vi "ProbeStationAutomation.vi"() -> ()   [LabVIEW 2020]
uses:
  Control 2.ctl
  C:/Users/User/Desktop/Automation/CurrentVersion/LabviewDXFViewer/bin/Release/LabviewDXFViewer.exe
  LabviewDXFViewer/bin/Release/LabviewDXFViewer.exe
  UIReferences.ctl
  WaferAlignmentType.ctl
  <vilib>/Utility/file.llb/Write Delimited Spreadsheet (DBL).vi
  Keithley 2600 Series/Keithley 2600 Series.lvlib
panel:
  in  "StartOxide":refnum<k24>(container)
  out "WaferAlignment":T1
  out "UiDefinition 3":T2
  in  "PathInfos":T3
  in  "UiDefinition 2":T2
  out "SweepInfo":T4
  out "error out":errorcluster
  out "Position 3":i32[](array[numeric])
  out "Position 2":i32[](array[numeric])
  out "Status":string="Please Load/Select probe site list"
  in  "Chip Orientation":i32(ring) items=["Horizontal", "Vertical"]
  in  "TextEditor":refnum<k24>(container)
  out "WaferTestPoints":string
  out "TestPointsLoaded":bool
  out "dxfFile":string
  out "error out 5":errorcluster
  out "Fit Array":string[][](array[string])
  out "error out 4":errorcluster
  out "error out 3":errorcluster
  out "Fit":dbl[][](array[numeric])
  out "IV Scan Data":dbl[][](array[numeric])
  out "Rotation Misalign":dbl[](array[numeric])
  out "Scale Misalign":dbl
  out "Position 1":i32[](array[numeric])
  in  "Microsites":refnum<k24>(container)
  in  "DXFCanvas":refnum<k24>(container)
  in  "WebCamViewer":refnum<k24>(container)
  in  "IV Curves":T5
  in  "Tab Control":T6(tab)
  in  "ClearPositions":bool
  in  "User":string
  in  "resetcontact":bool
  in  "EnableJoystick":bool
  in  "StartCycle":refnum<k24>(container)
  in  "Version":string
  in  "Experiment":string
  in  "Lower":refnum<k24>(container)
  in  "Raise":refnum<k24>(container)
  in  "West":refnum<k24>(container)
  in  "East":refnum<k24>(container)
  in  "North":refnum<k24>(container)
  in  "South":refnum<k24>(container)
  in  "Align Position 1":bool
  in  "Platten Move":refnum<k24>(container)
  in  "Masks":string(combo)
  in  "Move Position 1":bool
  in  "Align Position 3":bool
  in  "Position 3":bool
  in  "Align Position 2":bool
  in  "Position 2":bool
  in  "Die":string
  in  "Wafer":string
  in  "Jog (um) 2":dbl=100.0
  in  "Jog (um)":dbl=500.0
  in  "Load Mask":bool
  in  "Save Wafer":bool
  in  "Lift Distance (um)":dbl=2000.0
  in  "Quit":bool
  out "In Contact":bool
  out "Motor Position":string
  in  "Save Tag":string
  out "Capacitance":dbl
  in  "Current Range (A)":dbl=1e-10
  in  "Junction":string(combo)="None"
  in  "Sweeps":dbl=2.0
  in  "Number Points":dbl=200.0
  in  "Minimum (mV)":dbl=-100.0
  in  "Maxiumum (mV)":dbl=100.0
  in  "Source Measure Unit Channel (0: Channel A)":i32(ring) items=["Channel A", "Channel B"]
  in  "VISA resource name":refnum<visa-resource-name>="Keithley_2636A"
  in  "Scan":bool
  in  "Save Scan":bool
  out "Conductance":dbl
  out "Intercept":dbl
  out "XY Graph":cluster{"x":timestamp, "y":dbl}[](graph)
  in  "Steps Per micron":dbl=0.629
  in  "Stepper Controller Port":i32=3
  out "GetCameras":string[](array[string])
  in  "Wafer Definition File":path=path "C:/Users/User/Desktop/Automation/ASU FG Mask 21.08.26.dxf"
  in  "Wafer Units to microns":dbl=1.0
  in  "Data Path":path=path "C:/Users/User/Desktop/Automation/data"
  # "Run Oxide"
  # "Optional Tags"
  # "Jog Platten"
  # "Platten Altitude"
  # "Run IVs"
  # "Cycle Step"
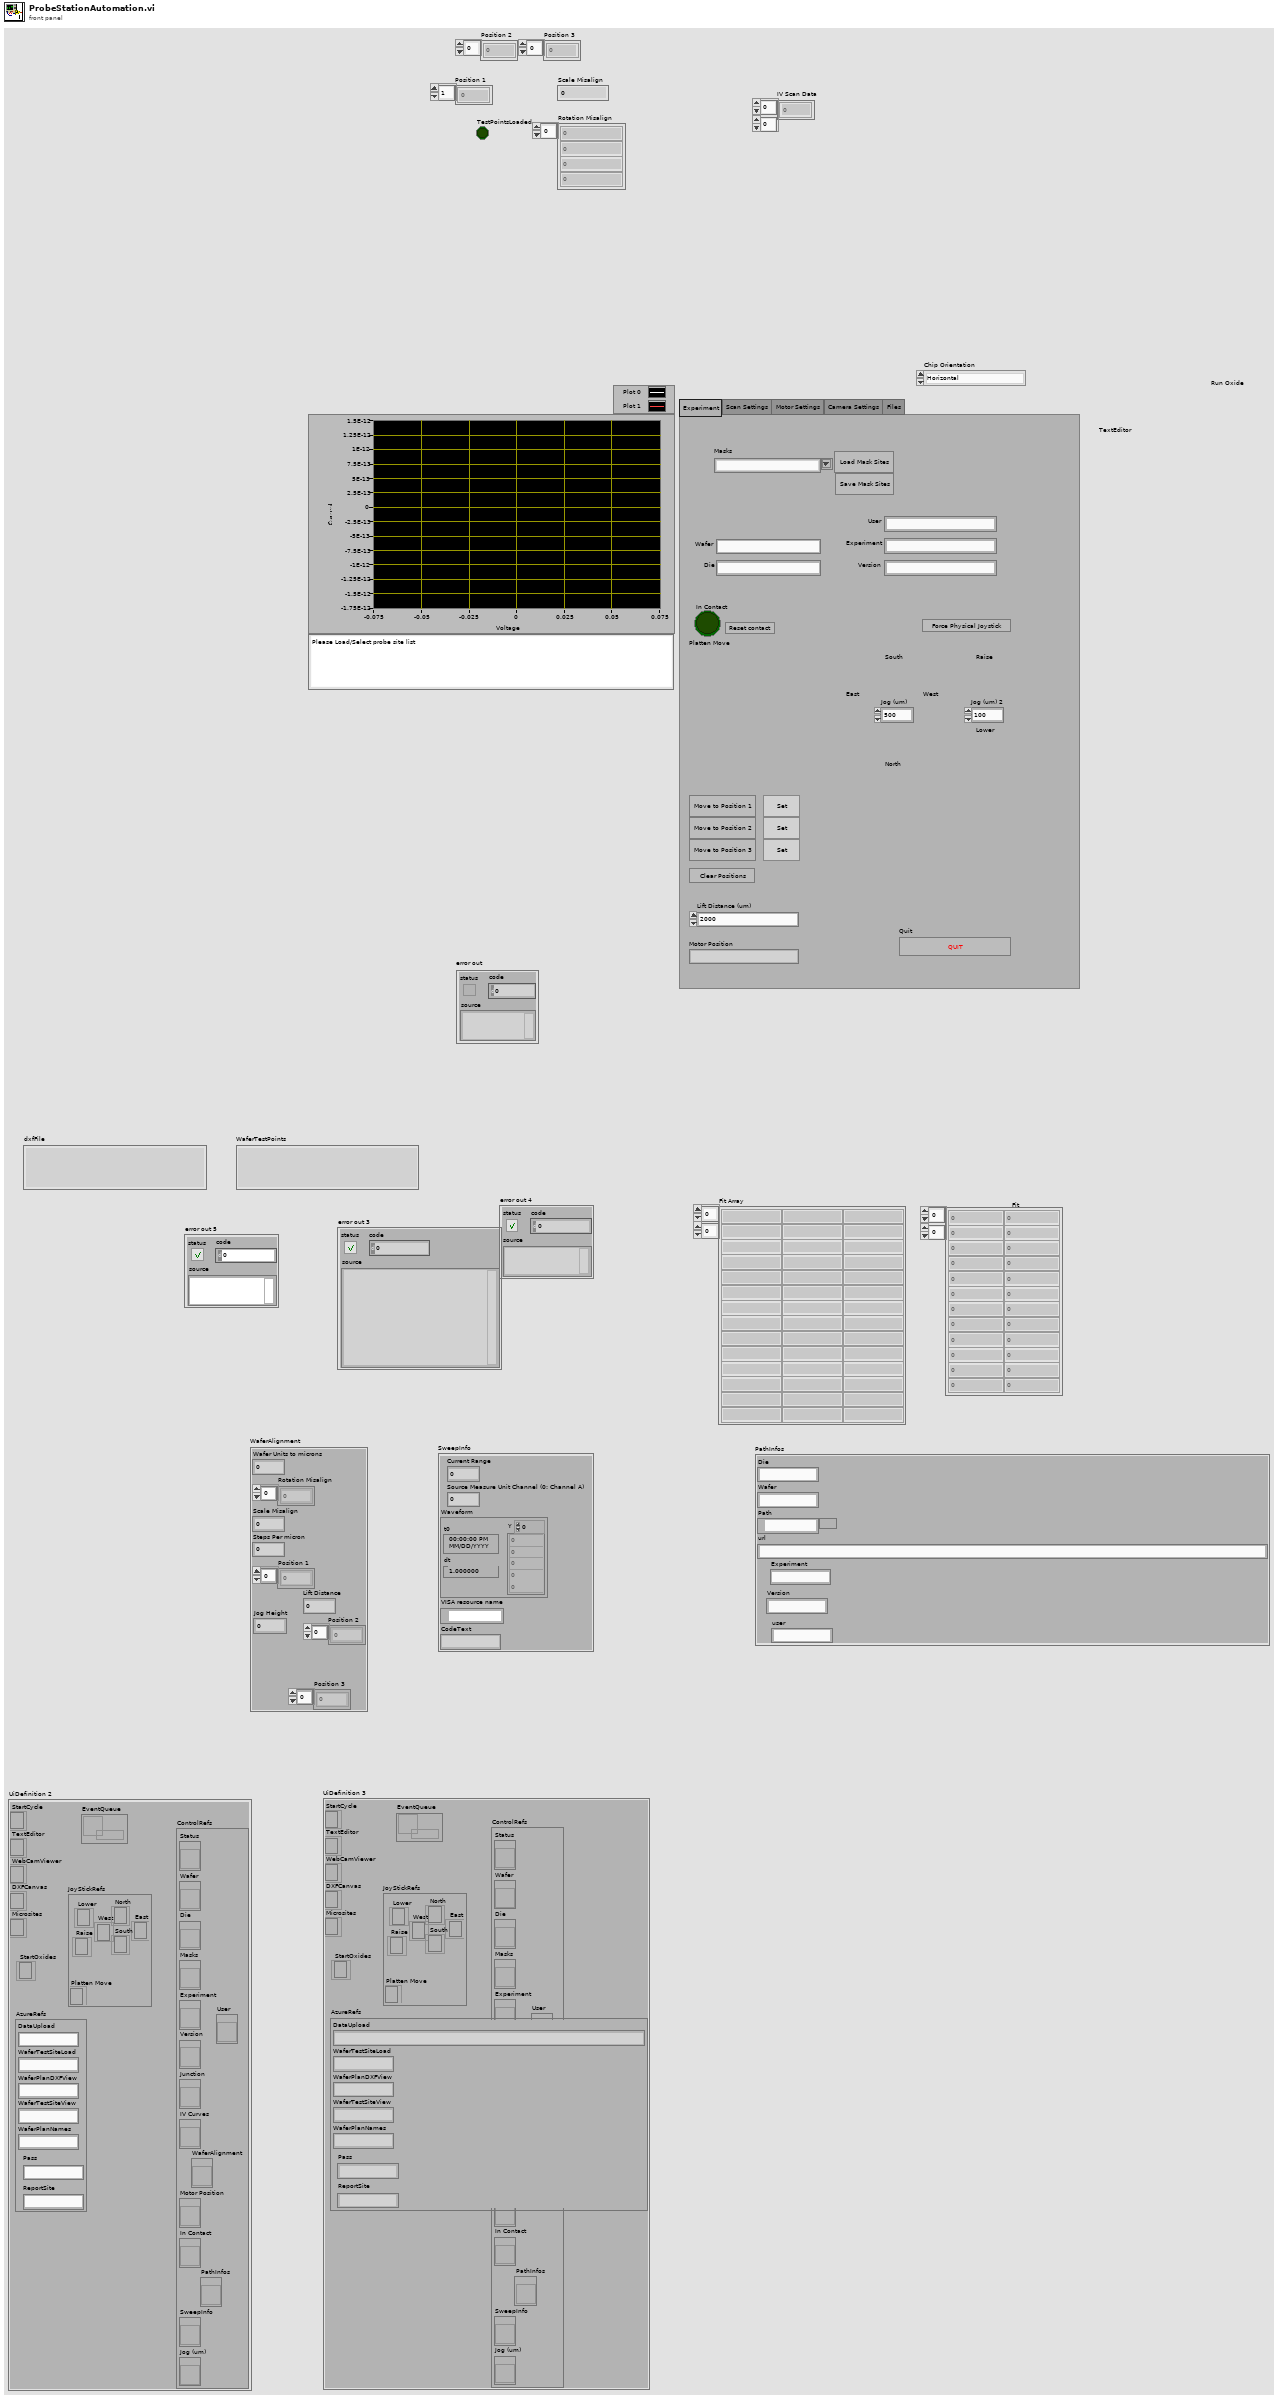
[diagram p1: front panel]
types:
  T1 = typedef "WaferAlignmentType.ctl" = cluster{"Wafer Units to microns":dbl, "Rotation Misalign":dbl[], "Scale Misalign":dbl, "Steps Per micron":dbl, "Position 1":i32[], "Position 2":i32[], "Lift Distance":i32, "Position 3":i32[], "Jog Height":i32}
  T2 = typedef "UIReferences.ctl" = cluster{"StartCycle":refnum<k24>, "TextEditor":refnum<k24>, "WebCamViewer":refnum<k24>, "DXFCanvas":refnum<k24>, "Microsites":refnum<k24>, "JoyStickRefs":cluster{"North":refnum<k24>, "Lower":refnum<k24>, "Raise":refnum<k24>, "Platten Move":refnum<k24>, "West":refnum<k24>, "East":refnum<k24>, "South":refnum<k24>}, "AzureRefs":cluster{"DataUpload":string, "WaferTestSiteLoad":string, "WaferPlanDXFView":string, "WaferTestSiteView":string, "WaferPlanNames":string, "Pass":string, "ReportSite":string}, "ControlRefs":cluster{"Status":refnum<vi>, "Wafer":refnum<vi>, "Die":refnum<vi>, "Masks":refnum<vi>, "Experiment":refnum<vi>, "Version":refnum<vi>, "Junction":refnum<vi>, "IV Curves":refnum<vi>, "Motor Position":refnum<vi>, "In Contact":refnum<vi>, "SweepInfo":refnum<vi>, "Jog (um)":refnum<vi>, "PathInfos":refnum<vi>, "User":refnum<vi>, "WaferAlignment":refnum<vi>}, "EventQueue":refnum<queue>, "StartOxides":refnum<k24>}
  T3 = cluster{"Die":string, "Wafer":string, "Path":path, "url":string, "Experiment":string, "Version":string, "user":string}
  T4 = cluster{"Current Range":dbl, "Source Measure Unit Channel (0: Channel A)":i32, "Waveform":waveform(dbl), "VISA resource name":refnum<visa-resource-name>, "CodeText":string}
  T5 = typedef "Control 2.ctl" = cluster{"Y":dbl[], "Current (A)":dbl[]}
  T6 = enum32{"Experiment", "Scan Settings", "Motor Settings", "Camera Settings", "Files"}
  T7 = cluster{"DataUpload":string, "WaferTestSiteLoad":string, "WaferPlanDXFView":string, "WaferTestSiteView":string, "WaferPlanNames":string, "Pass":string, "ReportSite":string}
  T8 = cluster{"North":refnum<k24>, "Lower":refnum<k24>, "Raise":refnum<k24>, "Platten Move":refnum<k24>, "West":refnum<k24>, "East":refnum<k24>, "South":refnum<k24>}
  T9 = cluster{"Status":refnum<vi>, "Wafer":refnum<vi>, "Die":refnum<vi>, "Masks":refnum<vi>, "Experiment":refnum<vi>, "Version":refnum<vi>, "Junction":refnum<vi>, "IV Curves":refnum<vi>, "Motor Position":refnum<vi>, "In Contact":refnum<vi>, "SweepInfo":refnum<vi>, "Jog (um)":refnum<vi>, "PathInfos":refnum<vi>, "User":refnum<vi>, "WaferAlignment":refnum<vi>}
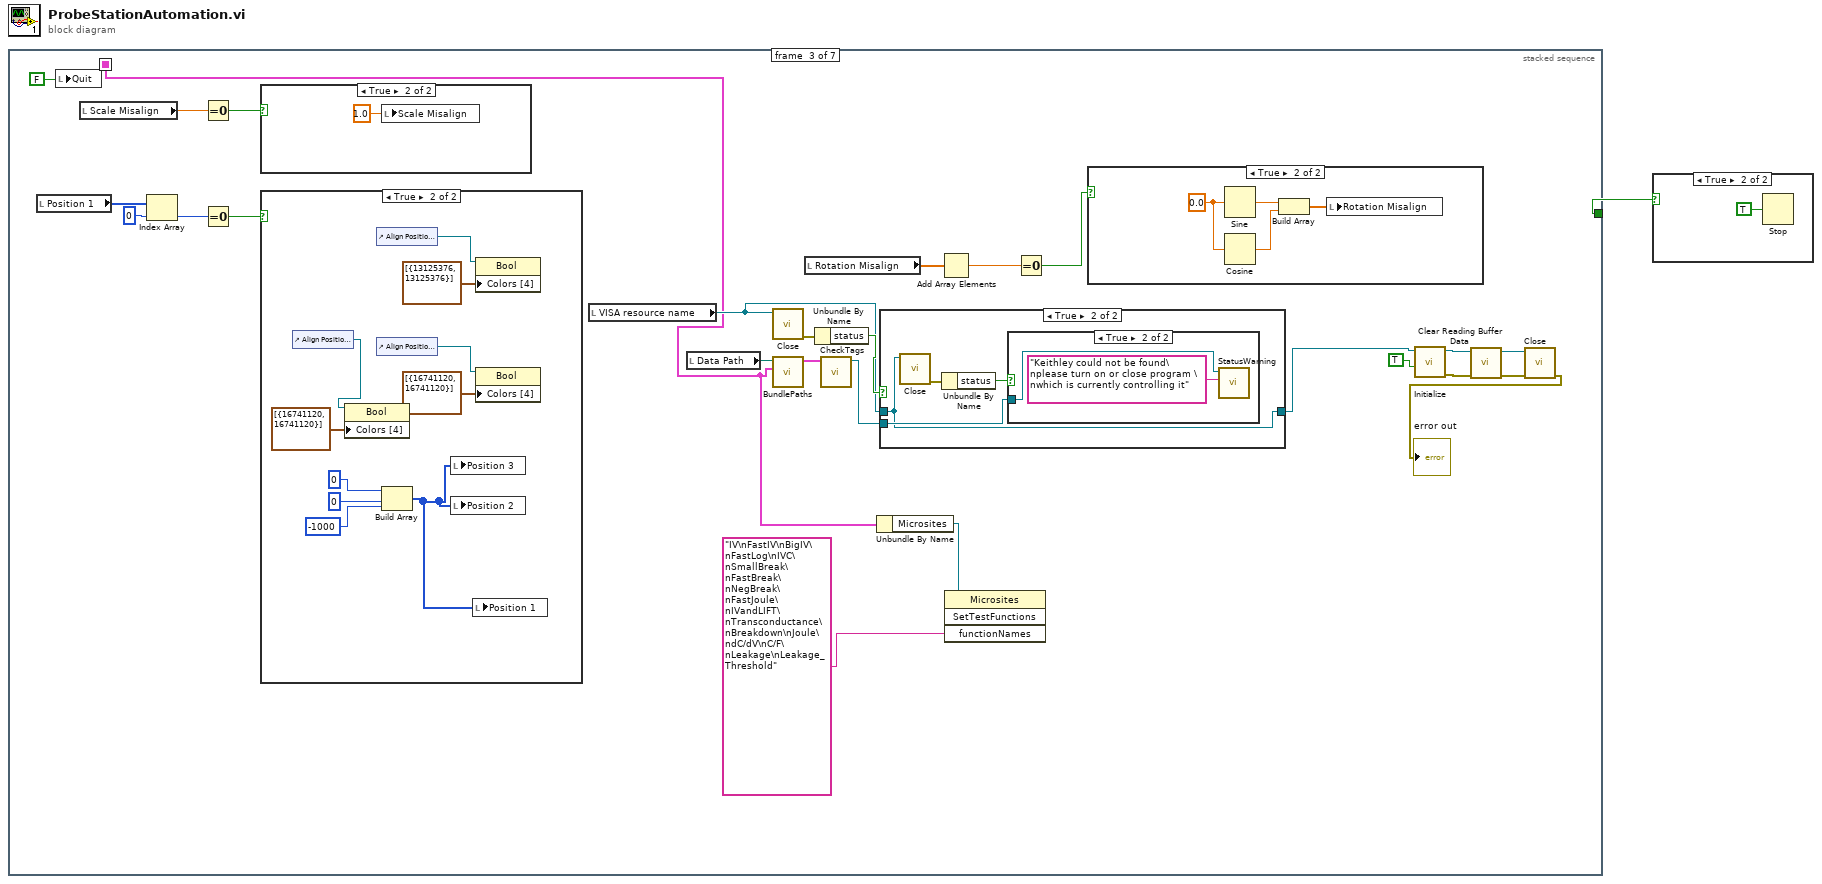
[diagram p0: block diagram]
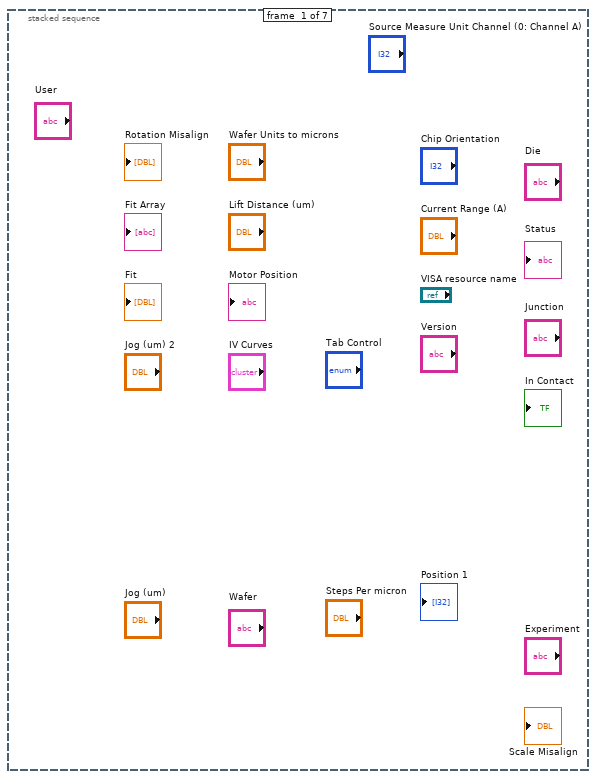
[diagram p3: hidden frame]
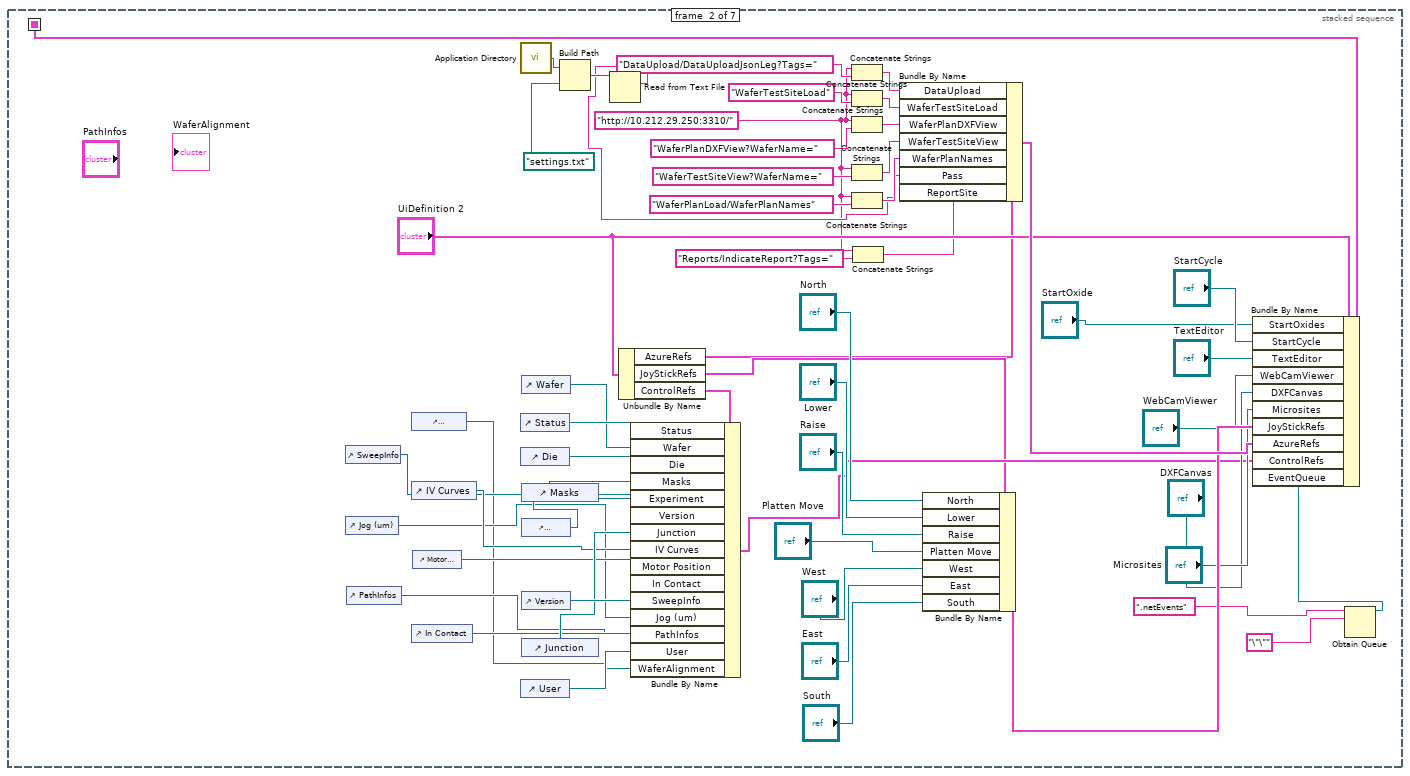
[diagram p4: hidden frame]
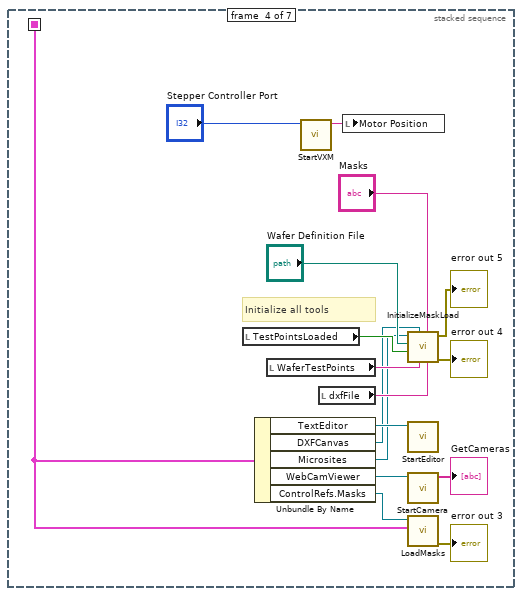
[diagram p10: hidden frame]
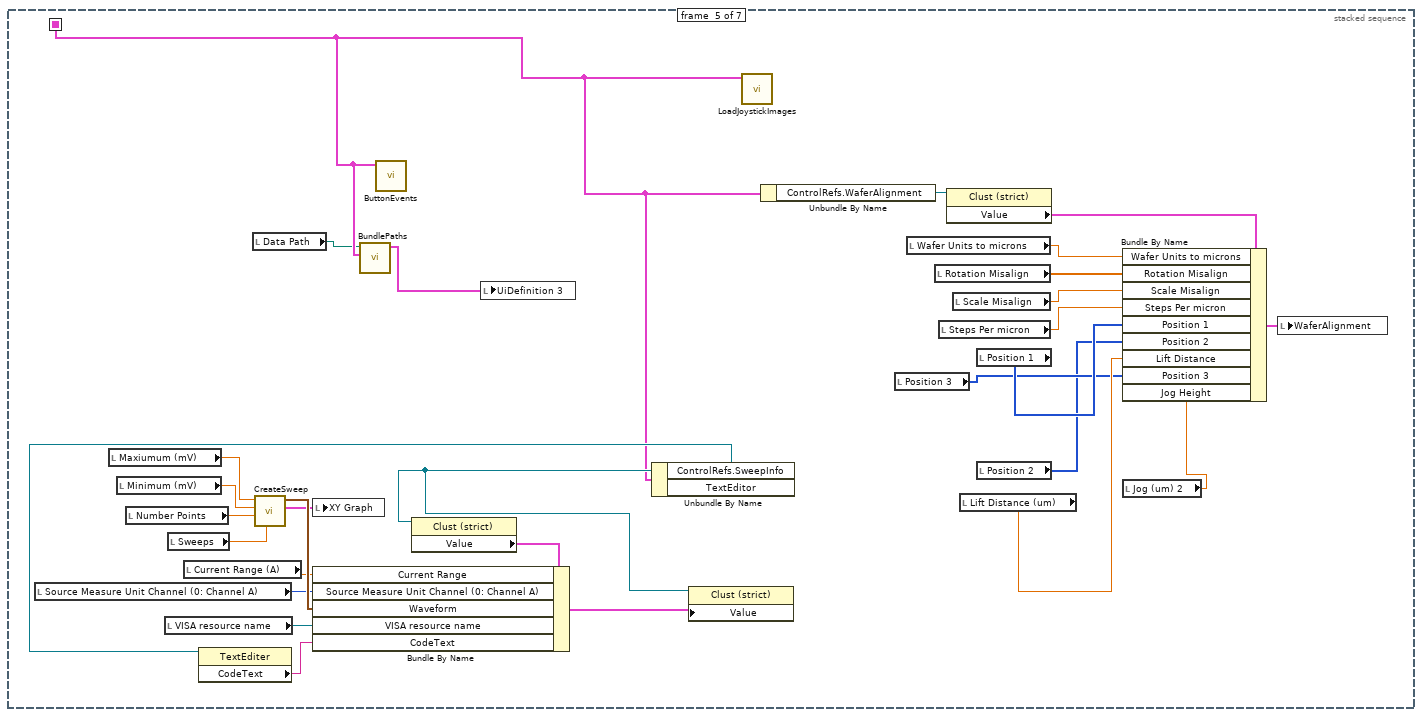
[diagram p11: hidden frame]
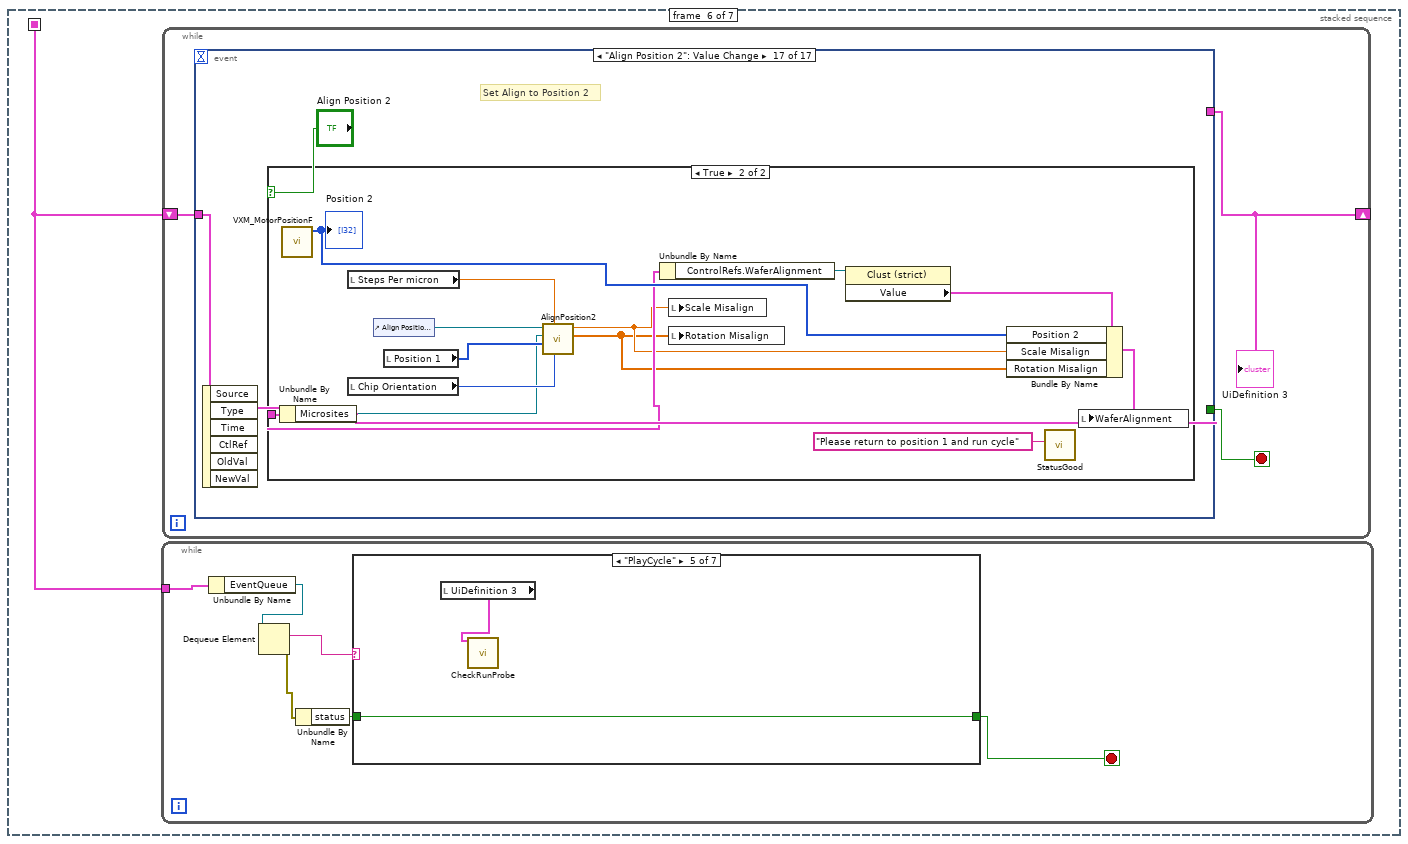
[diagram p12: hidden frame]
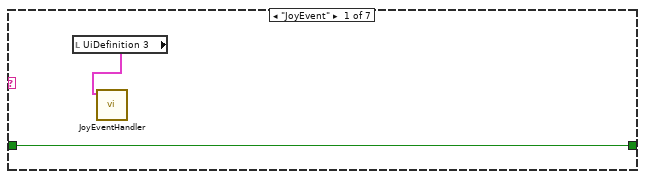
[diagram p13: hidden frame]
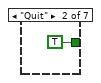
[diagram p14: hidden frame]
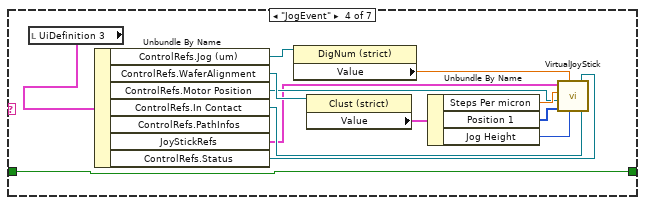
[diagram p16: hidden frame]
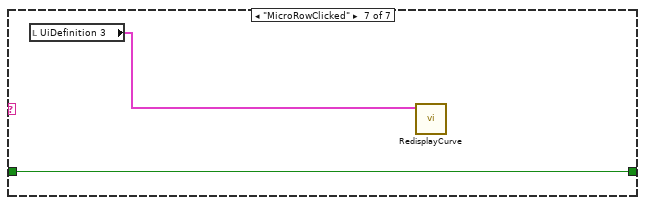
[diagram p18: hidden frame]
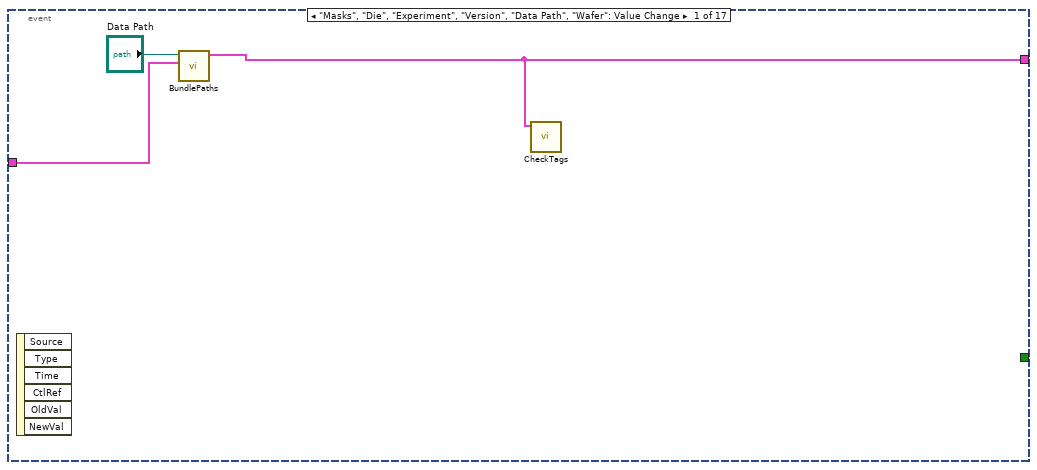
[diagram p19: hidden frame]
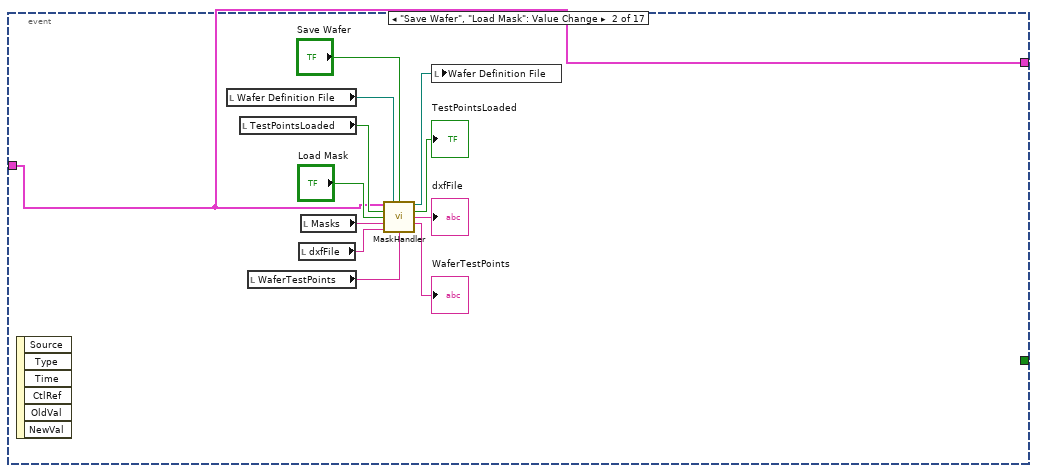
[diagram p20: hidden frame]
diagram:
  n1 = stacked-sequence {
    seq-local: [_ w44 _ _ _ _ _] -> [_ _ w60 w106 w125 w152 _]
    tunnel: [_ _ _ _ _ _ TRUE ("Quit")] -> w1
    frame #0 {
    }
    frame #1 {
      w3 = "http://10.212.29.250:3310/"
      n2 = control-ref of="SweepInfo"() -> (w29:refnum<vi>)
      n3 = control-ref of="Jog (um)"() -> (w28:refnum<vi>)
      n4 = control-ref of="PathInfos"() -> (w27:refnum<vi>)
      n5 = control-ref of="WaferAlignment"() -> (w5:refnum<vi>)
      n6 = control-ref of="IV Curves"() -> (w32:refnum<vi>)
      n7 = control-ref of="In Contact"() -> (w30:refnum<vi>)
      n8 = control-ref of="Motor Position"() -> (w31:refnum<vi>)
      n9 = call <vilib>:"Application Directory.vi"() -> ("Application Directory"=w8:path)
      n10 = control-ref of="Status"() -> (w39:refnum<vi>)
      n11 = control-ref of="Die"() -> (w37:refnum<vi>)
      n12 = control-ref of="User"() -> (w22:refnum<vi>)
      n13 = control-ref of="Wafer"() -> (w38:refnum<vi>)
      n14 = control-ref of="Masks"() -> (w36:refnum<vi>)
      n15 = control-ref of="Experiment"() -> (w35:refnum<vi>)
      n16 = control-ref of="Version"() -> (w34:refnum<vi>)
      n17 = control-ref of="Junction"() -> (w33:refnum<vi>)
      n18 = Build Path(base path=w8, name or relative path=path "settings.txt" ("file (use dialog)")) -> (appended path=w10:path)
      n19 = Read from Text File(file (use dialog)=w10) -> (text=w7:string)  [unwired: 3 in, 3 out]
      n20 = Unbundle By Name("UiDefinition 2") -> ("AzureRefs"=w21:T7, "JoyStickRefs"=w26:T8, "ControlRefs"=w41:T9)
      n21 = Bundle By Name(cluster=w41, "Status"=w39, "Wafer"=w38, "Die"=w37, "Masks"=w36, "Experiment"=w35, "Version"=w34, "Junction"=w33, "IV Curves"=w32, "Motor Position"=w31, "In Contact"=w30, "SweepInfo"=w29, "Jog (um)"=w28, "PathInfos"=w27, "User"=w22, "WaferAlignment"=w5) -> (w40:T9)
      n22 = Concatenate Strings(w3, "DataUpload/DataUploadJsonLeg?Tags=" ("url")) -> (w20:string)
      n23 = Concatenate Strings(w3, "WaferTestSiteLoad" ("url")) -> (w17:string)
      n24 = Concatenate Strings(w3, "WaferPlanDXFView?WaferName=" ("url")) -> (w15:string)
      n25 = Concatenate Strings(w3, "WaferTestSiteView?WaferName=" ("url")) -> (w13:string)
      n26 = Concatenate Strings(w3, "WaferPlanLoad/WaferPlanNames" ("url")) -> (w11:string)
      n27 = Concatenate Strings(w3, "Reports/IndicateReport?Tags=" ("string")) -> (w4:string)
      n28 = Bundle By Name(cluster=w21, "DataUpload"=w20, "WaferTestSiteLoad"=w17, "WaferPlanDXFView"=w15, "WaferTestSiteView"=w13, "WaferPlanNames"=w11, "Pass"=w7, "ReportSite"=w4) -> (w57:T7)
      n29 = Bundle By Name(cluster=w26, "North"="North", "Lower"="Lower", "Raise"="Raise", "Platten Move"="Platten Move", "West"="West", "East"="East", "South"="South") -> (w53:T8)
      n30 = Obtain Queue(name (unnamed)=".netEvents", element data type="\"\"") -> (queue out=w23:refnum<queue>)  [unwired: 3 in, 2 out]
      n31 = Bundle By Name(cluster="UiDefinition 2", "StartOxides"="StartOxide", "StartCycle"="StartCycle", "TextEditor"="TextEditor", "WebCamViewer"="WebCamViewer", "DXFCanvas"="DXFCanvas", "Microsites"="Microsites", "JoyStickRefs"=w53, "AzureRefs"=w57, "ControlRefs"=w40, "EventQueue"=w23) -> (w44:T2)
    }
    frame #2 {
      n32 = local read "Position 1"() -> (w82:i32[])
      n33 = local write "Quit"(FALSE) -> ()
      n34 = local read "Scale Misalign"() -> (w77:dbl)
      n35 = Index Array(array=w82, index=0) -> (element=w83:i32)
      n36 = Equal To 0?(x=w77) -> (x = 0?=w76:bool)
      n37 = Equal To 0?(x=w83) -> (x = 0?=w81:bool)
      n38 = case shown="True" w76 {
        frame False {
        }
        frame True {
          n39 = local write "Scale Misalign"(1.0 ("Scale Misalign")) -> ()
        }
      }
      n40 = case shown="True" w81 {
        frame False {
        }
        frame True {
          n41 = control-ref of="Align Position 3"() -> (w91:refnum<vi>)
          n42 = property class="Bool"(reference=w91, "Colors [4]"=cluster{u32, u32}[] [{16741120, 16741120}]) -> ()  [unwired: 1 in, 2 out]
          n43 = control-ref of="Align Position 1"() -> (w100:refnum<vi>)
          n44 = control-ref of="Align Position 2"() -> (w98:refnum<vi>)
          n45 = Build Array(0 ("Y"), 0 ("X"), -1000) -> (w93:i32[])
          n46 = local write "Position 3"(w93) -> ()
          n47 = local write "Position 2"(w93) -> ()
          n48 = local write "Position 1"(w93) -> ()
          n49 = property class="Bool"(reference=w100, "Colors [4]"=cluster{u32, u32}[] [{13125376, 13125376}]) -> ()  [unwired: 1 in, 2 out]
          n50 = property class="Bool"(reference=w98, "Colors [4]"=cluster{u32, u32}[] [{16741120, 16741120}]) -> ()  [unwired: 1 in, 2 out]
        }
      }
      n51 = local read "VISA resource name"() -> (w69:refnum<visa-resource-name>)
      n52 = local read "Data Path"() -> (w66:path)
      n53 = call "Close.vi"("VISA resource name"=w69) -> ("error out"=w73:errorcluster)  [unwired: 10 in]
      n54 = call "BundlePaths.vi"("Data Path"=w66, "UiDefinition 2"=w60) -> ("UiDefinition 3"=w67:T2)  [unwired: 8 in]
      n55 = local read "Rotation Misalign"() -> (w80:dbl[])
      n56 = Unbundle By Name(w73) -> ("status"=w72:bool)
      n57 = call "CheckTags.vi"("UiDefinition 2"=w67) -> ("StatusOut"=w71:refnum<vi>)  [unwired: 10 in]
      n58 = Unbundle By Name(w60) -> ("Microsites"=w59:refnum<k24>)
      n59 = case shown="True" w72 {
        tunnel: w71 -> [_ w88]
        tunnel: w69 -> [w84 w87]
        tunnel: [w84 w87] -> w68
        frame False {
        }
        frame True {
          n60 = call "Close.vi"("VISA resource name"=w87) -> ("error out"=w86:errorcluster)  [unwired: 10 in]
          n61 = Unbundle By Name(w86) -> ("status"=w85:bool)
          n62 = case shown="True" w85 {
            tunnel: w88 -> [_ w89]
            frame False {
            }
            frame True {
              n63 = call "StatusWarning.vi"("Text.Text"="Keithley could not be found\nplease turn on or close program \nwhich is currently controlling it", "String in"=w89) -> ()  [unwired: 10 in]
            }
          }
        }
      }
      n64 = Add Array Elements(numeric array=w80) -> (sum=w79:dbl)
      n65 = invoke class="Microsites" method="SetTestFunctions"(reference=w59, "functionNames"="IV\nFastIV\nBigIV\nFastLog\nIVC\nSmallBreak\nFastBreak\nNegBreak\nFastJoule\nIVandLIFT\nTransconductance\nBreakdown\nJoule\ndC/dV\nC/F\nLeakage\nLeakage_Threshold") -> ()  [unwired: 2 in, 4 out]
      n66 = Equal To 0?(x=w79) -> (x = 0?=w78:bool)
      n67 = case shown="True" w78 {
        frame False {
        }
        frame True {
          w101 = 0.0 ("x")
          n68 = Sine(x=w101) -> (sin(x)=w104:dbl)
          n69 = Cosine(x=w101) -> (cos(x)=w103:dbl)
          n70 = Build Array(w104, w103) -> (w102:dbl[])
          n71 = local write "Rotation Misalign"(w102) -> ()
        }
      }
      n72 = call "Initialize.vi"("Reset (True)"=TRUE, "VISA resource name"=w68) -> ("error out"=w64:errorcluster, "VISA resource name out"=w65:refnum<visa-resource-name>)  [unwired: 8 in]
      n73 = call "Clear Reading Buffer Data.vi"("error in (no error)"=w64, "VISA resource name"=w65) -> ("error out"=w63:errorcluster, "VISA resource name out"=w62:refnum<visa-resource-name>)  [unwired: 8 in]
      n74 = call "Close.vi"("error in (no error)"=w63, "VISA resource name"=w62) -> ("error out"=→"error out":errorcluster)  [unwired: 9 in]
    }
    frame #3 {
      # "Initialize all tools"
      n75 = local read "TestPointsLoaded"() -> (w117:bool)
      n76 = Unbundle By Name(w106) -> ("TextEditor"=w111:refnum<k24>, "DXFCanvas"=w110:refnum<k24>, "Microsites"=w109:refnum<k24>, "WebCamViewer"=w108:refnum<k24>, "ControlRefs.Masks"=w107:refnum<vi>)
      n77 = local read "WaferTestPoints"() -> (w116:string)
      n78 = call "StartVXM.vi"("Stepper Controller Port"="Stepper Controller Port") -> ("String"=w112:string)  [unwired: 10 in]
      n79 = local read "dxfFile"() -> (w115:string)
      n80 = local write "Motor Position"(w112) -> ()
      n81 = call "InitializeMaskLoad.vi"("dxfFile"=w115, "Masks"="Masks", "WaferTestPoints"=w116, "DXFCanvas"=w110, "TestPointsLoaded"=w117, "Wafer Definition File"="Wafer Definition File", "MicrositesRef"=w109) -> ("error out"=→"error out 4":errorcluster, "error out 5"=→"error out 5":errorcluster)  [unwired: 3 in]
      n82 = call "StartEditor.vi"("CodeEditorRef"=w111) -> ()  [unwired: 11 in]
      n83 = call "StartCamera.vi"("WebCamViewerRef"=w108) -> ("GetCameras"=→"GetCameras":string[])  [unwired: 10 in]
      n84 = call "LoadMasks.vi"("UiDefinition 2"=w106, "ComboBox in"=w107) -> ("error out"=→"error out 3":errorcluster)  [unwired: 9 in]
    }
    frame #4 {
      n85 = local read "Source Measure Unit Channel (0: Channel A)"() -> (w134:i32)
      n86 = local read "Maxiumum (mV)"() -> (w131:dbl)
      n87 = local read "Minimum (mV)"() -> (w130:dbl)
      n88 = local read "Number Points"() -> (w129:dbl)
      n89 = local read "VISA resource name"() -> (w139:refnum<visa-resource-name>)
      n90 = local read "Sweeps"() -> (w128:dbl)
      n91 = local read "Current Range (A)"() -> (w133:dbl)
      n92 = local read "Data Path"() -> (w123:path)
      n93 = call "CreateSweep.vi"("Sweeps"=w128, "Number Points"=w129, "Minimum Voltage"=w130, "Maxiumum Voltage"=w131) -> ("XY pairs"=w127:cluster{"x":timestamp, "y":dbl}[], "Waveform"=w135:waveform(dbl))  [unwired: 6 in]
      n94 = local write "XY Graph"(w127) -> ()
      n95 = call "BundlePaths.vi"("Data Path"=w123, "UiDefinition 2"=w125) -> ("UiDefinition 3"=w124:T2)  [unwired: 8 in]
      n96 = call "ButtonEvents.vi"("UiDefinition"=w125) -> ()  [unwired: 11 in]
      n97 = local write "UiDefinition 3"(w124) -> ()
      n98 = Unbundle By Name(w125) -> ("ControlRefs.SweepInfo"=w137:refnum<vi>, "TextEditor"=w138:refnum<k24>)
      n99 = property class="TextEditer"(reference=w138) -> ("CodeText"=w140:string)  [unwired: 1 in, 2 out]
      n100 = property class="Clust (strict)"(reference=w137) -> ("Value"=w136:T4)  [unwired: 1 in, 2 out]
      n101 = Bundle By Name(cluster=w136, "Current Range"=w133, "Source Measure Unit Channel (0: Channel A)"=w134, "Waveform"=w135, "VISA resource name"=w139, "CodeText"=w140) -> (w132:T4)
      n102 = property class="Clust (strict)"(reference=w137, "Value"=w132) -> ()  [unwired: 1 in, 2 out]
      n103 = call "LoadJoystickImages.vi"("UiDefinition 2"=w125) -> ()  [unwired: 11 in]
      n104 = Unbundle By Name(w125) -> ("ControlRefs.WaferAlignment"=w151:refnum<vi>)
      n105 = local read "Position 3"() -> (w143:i32[])
      n106 = local read "Wafer Units to microns"() -> (w148:dbl)
      n107 = local read "Rotation Misalign"() -> (w147:dbl[])
      n108 = local read "Steps Per micron"() -> (w141:dbl)
      n109 = property class="Clust (strict)"(reference=w151) -> ("Value"=w150:T1)  [unwired: 1 in, 2 out]
      n110 = local read "Scale Misalign"() -> (w146:dbl)
      n111 = local read "Lift Distance (um)"() -> (w144:dbl)
      n112 = local read "Position 1"() -> (w145:i32[])
      n113 = local read "Position 2"() -> (w142:i32[])
      n114 = local read "Jog (um) 2"() -> (w126:dbl)
      n115 = Bundle By Name(cluster=w150, "Wafer Units to microns"=w148, "Rotation Misalign"=w147, "Scale Misalign"=w146, "Steps Per micron"=w141, "Position 1"=w145, "Position 2"=w142, "Lift Distance"=w144, "Position 3"=w143, "Jog Height"=w126) -> (w149:T1)
      n116 = local write "WaferAlignment"(w149) -> ()
    }
    frame #5 {
      n117 = while {
        tunnel: w152 -> [w153]
        stop <- w154 stop-if-true
        n118 = Unbundle By Name(w153) -> ("EventQueue"=w157:refnum<queue>)
        n119 = Dequeue Element(queue=w157) -> (element=w158:string, error out=w156:errorcluster)  [unwired: 2 in, 2 out]
        n120 = Unbundle By Name(w156) -> ("status"=w155:bool)
        n121 = case shown="\"PlayCycle\"" w158 {
          tunnel: w155 -> [w160 _ w162 w164 w177 w178 w180]
          tunnel: [w160 TRUE ("status") w162 w164 w177 w178 w180] -> w154
          frame "JoyEvent" {
            n122 = local read "UiDefinition 3"() -> (w159:T2)
            n123 = call "JoyEventHandler.vi"("UiDefinition"=w159) -> ()  [unwired: 11 in]
          }
          frame "Quit" {
          }
          frame Default {
          }
          frame "JogEvent" {
            n124 = local read "UiDefinition 3"() -> (w163:T2)
            n125 = Unbundle By Name(w163) -> ("ControlRefs.Jog (um)"=w167:refnum<vi>, "ControlRefs.WaferAlignment"=w175:refnum<vi>, "ControlRefs.Motor Position"=w172:refnum<vi>, "ControlRefs.In Contact"=w170:refnum<vi>, "JoyStickRefs"=w168:T8, "ControlRefs.Status"=w165:refnum<vi>)  [unwired: 1 out]
            n126 = property class="DigNum (strict)"(reference=w167) -> ("Value"=w166:dbl)  [unwired: 1 in, 2 out]
            n127 = property class="Clust (strict)"(reference=w175) -> ("Value"=w174:T1)  [unwired: 1 in, 2 out]
            n128 = Unbundle By Name(w174) -> ("Steps Per micron"=w173:dbl, "Position 1"=w171:i32[], "Jog Height"=w169:i32)
            n129 = call "VirtualJoyStick.vi"("In Contact"=w170, "Status"=w165, "Jog (um) raise"=w169, "Jog (um)"=w166, "Position 1"=w171, "Motor Zero"=w172, "Steps Per micron"=w173, "JoyStickRefs"=w168) -> ()
          }
          frame "PlayCycle" {
            n130 = local read "UiDefinition 3"() -> (w176:T2)
            n131 = call "CheckRunProbe.vi"("UiDefinition"=w176) -> ()  [unwired: 15 in]
          }
          frame "OxideCycle" {
          }
          frame "MicroRowClicked" {
            n132 = local read "UiDefinition 3"() -> (w179:T2)
            n133 = call "RedisplayCurve.vi"("UiDefinition 3"=w179) -> ()  [unwired: 11 in]
          }
        }
      }
      n134 = while {
        shift-right: [w182] -> _
        shift-left: w152 -> [w183]
        stop <- w181 stop-if-true
        n135 = event shown="[16] \"Align Position 2\": Value Change" {
          selector: _ -> [_ _ _ _ _ _ _ _ _ _ _ _ _ _ _ _ _]
          dyn-events: _ -> [_ _ _ _ _ _ _ _ _ _ _ _ _ _ _ _ _]
          timeout: _ -> [_ _ _ _ _ _ _ _ _ _ _ _ _ _ _ _ _]
          tunnel: w183 -> [w185 w187 w199 w206 w223 w229 w238 w247 w255 w259 w263 w327 w329 w345 w349 w359 w371]
          tunnel: [w184 w187 w199 w206 w223 w229 w238 w247 w255 w259 w263 w327 w329 w345 w349 w359 w371] -> w182
          tunnel: [_ _ _ _ _ _ "Quit" _ _ _ _ _ _ _ _ _ _] -> w181
          event "Masks", "Die", "Experiment", "Version", "Data Path", "Wafer": Value Change {
            n136 = event-data() -> ()  [unwired: 1 in, 6 out]
            n137 = call "BundlePaths.vi"("Data Path"="Data Path", "UiDefinition 2"=w185) -> ("UiDefinition 3"=w184:T2)  [unwired: 8 in]
            n138 = call "CheckTags.vi"("UiDefinition 2"=w184) -> ()  [unwired: 10 in, 1 out]
          }
          event "Save Wafer", "Load Mask": Value Change {
            n139 = event-data() -> ()  [unwired: 1 in, 6 out]
            n140 = local read "Wafer Definition File"() -> (w195:path)
            n141 = local read "TestPointsLoaded"() -> (w192:bool)
            n142 = local read "WaferTestPoints"() -> (w196:string)
            n143 = local read "dxfFile"() -> (w198:string)
            n144 = local read "Masks"() -> (w189:string)
            n145 = call "MaskHandler.vi"("UiDefinition 2"=w187, "Wafer Definition File"=w195, "Save Wafer"="Save Wafer", "TestPointsLoaded in"=w192, "Load Mask"="Load Mask", "Masks"=w189, "dxfFile"=w198, "WaferTestPoints"=w196) -> ("Path"=w193:path, "TestPointsLoaded out"=→"TestPointsLoaded":bool, "body 2"=→"dxfFile":string, "body"=→"WaferTestPoints":string)  [unwired: 4 in]
            n146 = local write "Wafer Definition File"(w193) -> ()
          }
          event "Scan": Value Change {
            # "On request IV curve"
            n147 = event-data() -> ()  [unwired: 1 in, 6 out]
            n148 = case shown="True" "Scan" {
              tunnel: w199 -> [_ w202]
              frame False {
              }
              frame True {
                n149 = call "SingleIV.vi"("UiDefinition 2"=w202) -> ("appended array"=→"IV Scan Data":dbl[][], "CapacitanceIV"=→"Capacitance":dbl, "slope"=→"Conductance":dbl, "intercept"=→"Intercept":dbl)  [unwired: 11 in]
              }
            }
          }
          event "Align Position 1": Value Change {
            n150 = event-data() -> ()  [unwired: 1 in, 6 out]
            n151 = Unbundle By Name(w206) -> ("ControlRefs.Status"=w207:refnum<vi>)
            n152 = case shown="True" "Align Position 1" {
              tunnel: w207 -> [_ w215]
              tunnel: w206 -> [_ w210]
              frame False {
              }
              frame True {
                n153 = Unbundle By Name(w210) -> ("ControlRefs.WaferAlignment"=w213:refnum<vi>)
                n154 = local write "In Contact"(TRUE) -> ()
                n155 = property class="Clust (strict)"(reference=w213) -> ("Value"=w212:T1)  [unwired: 1 in, 2 out]
                n156 = control-ref of="Align Position 1"() -> (w218:refnum<vi>)
                n157 = call "VXM_MotorPositionF.vi"() -> ("Position"=w211:i32[])  [unwired: 11 in]
                n158 = Bundle By Name(cluster=w212, "Position 1"=w211) -> (w209:T1)
                n159 = local write "Position 1"(w211) -> ()
                n160 = property class="Bool"(reference=w218, "Colors [4]"=cluster{u32, u32}[] [{13816530, 13816530}]) -> ()  [unwired: 1 in, 2 out]
                n161 = local write "WaferAlignment"(w209) -> ()
                n162 = call "StatusGood.vi"("Text.Text"="Align Position 2 or run cycle" ("Status"), "String in"=w215) -> ()  [unwired: 10 in]
              }
            }
          }
          event "Minimum (mV)", "Maxiumum (mV)", "Number Points", "Sweeps": Value Change {
            n163 = event-data() -> ()  [unwired: 1 in, 6 out]
            n164 = Unbundle By Name(w223) -> ("ControlRefs.SweepInfo"=w219:refnum<vi>)
            n165 = call "CreateSweep.vi"("Sweeps"="Sweeps", "Number Points"="Number Points", "Minimum Voltage"="Minimum (mV)", "Maxiumum Voltage"="Maxiumum (mV)") -> ("XY pairs"=→"XY Graph":cluster{"x":timestamp, "y":dbl}[], "Waveform"=w221:waveform(dbl))  [unwired: 6 in]
            n166 = property class="Clust (strict)"(reference=w219) -> ("Value"=w222:T4)  [unwired: 1 in, 2 out]
            n167 = Bundle By Name(cluster=w222, "Waveform"=w221) -> (w220:T4)
            n168 = property class="Clust (strict)"(reference=w219, "Value"=w220) -> ()  [unwired: 1 in, 2 out]
          }
          event "Current Range (A)", "VISA resource name", "Source Measure Unit Channel (0: Channel A)": Value Change {
            n169 = event-data() -> ()  [unwired: 1 in, 6 out]
            n170 = Unbundle By Name(w229) -> ("ControlRefs.SweepInfo"=w232:refnum<vi>, "TextEditor"=w233:refnum<k24>)
            n171 = local read "Source Measure Unit Channel (0: Channel A)"() -> (w234:i32)
            n172 = local read "VISA resource name"() -> (w235:refnum<visa-resource-name>)
            n173 = local read "Current Range (A)"() -> (w236:dbl)
            n174 = property class="Clust (strict)"(reference=w232) -> ("Value"=w230:T4)  [unwired: 1 in, 2 out]
            n175 = property class="TextEditer"(reference=w233) -> ("CodeText"=w237:string)  [unwired: 1 in, 2 out]
            n176 = Bundle By Name(cluster=w230, "Current Range"=w236, "Source Measure Unit Channel (0: Channel A)"=w234, "VISA resource name"=w235, "CodeText"=w237) -> (→"SweepInfo":T4)
          }
          event "Quit": Value Change {
            n177 = event-data() -> ()  [unwired: 1 in, 6 out]
            n178 = Unbundle By Name(w238) -> ("EventQueue"=w240:refnum<queue>)
            n179 = Enqueue Element(queue=w240, element="Quit") -> ()  [unwired: 2 in, 3 out]
          }
          event "Position 1", "Wafer Units to microns", "Rotation Misalign", "Scale Misalign", "Steps Per micron", "Lift Distance (um)", "Jog (um) 2": Value Change {
            n180 = event-data() -> ()  [unwired: 1 in, 6 out]
            n181 = Unbundle By Name(w247) -> ("ControlRefs.WaferAlignment"=w249:refnum<vi>)
            n182 = property class="Clust (strict)"(reference=w249) -> ("Value"=w248:T1)  [unwired: 1 in, 2 out]
            n183 = local read "Wafer Units to microns"() -> (w253:dbl)
            n184 = local read "Rotation Misalign"() -> (w250:dbl[])
            n185 = local read "Lift Distance (um)"() -> (w244:dbl)
            n186 = local read "Steps Per micron"() -> (w251:dbl)
            n187 = local read "Scale Misalign"() -> (w252:dbl)
            n188 = local read "Jog (um) 2"() -> (w243:dbl)
            n189 = local read "Position 1"() -> (w254:i32[])
            n190 = local read "Position 2"() -> (w246:i32[])
            n191 = local read "Position 3"() -> (w245:i32[])
            n192 = Bundle By Name(cluster=w248, "Wafer Units to microns"=w253, "Rotation Misalign"=w250, "Scale Misalign"=w252, "Steps Per micron"=w251, "Position 1"=w254, "Position 2"=w246, "Lift Distance"=w244, "Position 3"=w245, "Jog Height"=w243) -> (w242:T1)
            n193 = local write "WaferAlignment"(w242) -> ()
          }
          event "Move Position 1": Value Change {
            n194 = event-data() -> ()  [unwired: 1 in, 6 out]
            n195 = local read "In Contact"() -> (w258:bool)
            n196 = call "MovePos1.vi"("In Contact in"=w258, "Move Position 1"="Move Position 1", "UiDefinition 2"=w255) -> ("In Contact out"=w257:bool)  [unwired: 8 in]
            n197 = local write "In Contact"(w257) -> ()
          }
          event "Position 2": Value Change {
            n198 = event-data() -> ()  [unwired: 1 in, 6 out]
            n199 = local read "In Contact"() -> (w262:bool)
            n200 = call "MoveToPosition2.vi"("In Contact in"=w262, "Position in"="Position 2", "UiDefinition 2"=w259) -> ("In Contact out"=w261:bool)  [unwired: 8 in]
            n201 = local write "In Contact"(w261) -> ()
          }
          event "Save Scan": Value Change {
            n202 = event-data() -> ()  [unwired: 1 in, 6 out]
            n203 = case shown="True" "Save Scan" {
              tunnel: w263 -> [_ w271]
              frame False {
              }
              frame True {
                n204 = Unbundle By Name(w271) -> ("ControlRefs.PathInfos"=w274:refnum<vi>)  [unwired: 1 out]
                n205 = local read "Junction"() -> (w268:string)
                n206 = property class="Clust (strict)"(reference=w274) -> ("Value"=w273:T3)  [unwired: 1 in, 2 out]
                n207 = Not Equal?(x="None", y=w268) -> (x != y?=w270:bool)
                n208 = local read "IV Scan Data"() -> (w277:dbl[][])
                n209 = Unbundle By Name(w273) -> ("Path"=w266:path, "url"=w272:string)
                n210 = call <vilib>:"Check if File or Folder Exists.vi"("path"=w266) -> ("file or folder exists?"=w267:bool)  [unwired: 8 in, 2 out]
                n211 = case shown="False" w267 {
                  tunnel: w266 -> [w279 w280]
                  tunnel: [w278 w280] -> w265
                  frame False {
                    n212 = Create Folder(path (use dialog)=w279) -> (created path=w278:path)  [unwired: 2 in, 2 out]
                  }
                  frame True {
                  }
                }
                n213 = case shown="True" TRUE {
                  tunnel: w277 -> [_ w289]
                  tunnel: "Save Tag" -> [_ w283]
                  tunnel: w270 -> [_ w285]
                  tunnel: w268 -> [_ w282]
                  tunnel: w265 -> [_ w281]
                  frame False {
                  }
                  frame True {
                    n214 = Empty String/Path?(string/path=w283) -> (empty?=w284:bool)
                    n215 = case shown="True" w285 {
                      tunnel: [w293 FALSE ("cancelled")] -> w288
                      tunnel: [w292 w294] -> w287
                      tunnel: [w291 errorcluster {"status"=FALSE, "code"=0, "source"=""} ("error out")] -> w286
                      tunnel: w284 -> [_ w298]
                      tunnel: w281 -> [w290 w297]
                      tunnel: w283 -> [_ w296]
                      tunnel: w282 -> [_ w295]
                      frame False {
                        n216 = call "File Dialog"("start path"=w290) -> ("selected path"=w292:path, "cancelled"=w293:bool, "error out"=w291:errorcluster)  [unwired: 11 in, 1 out]
                      }
                      frame True {
                        n217 = case shown="True" w298 {
                          tunnel: w297 -> [w307 w311]
                          tunnel: [w306 w312] -> w294
                          tunnel: w296 -> [w302 _]
                          tunnel: w295 -> [w304 w310]
                          frame False {
                            n218 = Concatenate Strings(w304, "_" ("string"), w302, ".csv" ("string")) -> (w305:string)
                            n219 = Build Path(base path=w307, name or relative path=w305) -> (appended path=w306:path)
                          }
                          frame True {
                            n220 = Concatenate Strings(w310, "_m.csv" ("string")) -> (w309:string)
                            n221 = Build Path(base path=w311, name or relative path=w309) -> (appended path=w312:path)
                          }
                        }
                      }
                    }
                    n222 = case shown="False" w288 {
                      tunnel: w289 -> [w314 _]
                      tunnel: w287 -> [w313 _]
                      tunnel: w286 -> [_ _]
                      frame False {
                        n223 = call-poly <vilib>:"Write Delimited Spreadsheet.vi"("file path (dialog if empty)"=w313, "format (%.3f)"="%.9e", "2D data"=w314, "transpose? (no:F)"=TRUE, "delimiter (\\t)"="," ("delimiter (\\t)")) -> ()  [unwired: 9 in, 2 out]
                      }
                      frame True {
                      }
                    }
                  }
                }
                n224 = case shown="True" w270 {
                  tunnel: w277 -> [_ w326]
                  tunnel: w272 -> [_ w324]
                  tunnel: w268 -> [_ w323]
                  tunnel: w271 -> [_ w321]
                  tunnel: "Save Tag" -> [_ w319]
                  frame False {
                  }
                  frame True {
                    n225 = Concatenate Strings(w319, "|" ("string"), w323) -> (w320:string)
                    n226 = Search and Replace String(input string=w324, search string="JuncName" ("string"), replace string=w320) -> (result string=w325:string)  [unwired: 5 in, 3 out]
                    n227 = call "UploadIV.vi"("UiDefinition 2"=w321, "IV Scan Data"=w326, "url"=w325) -> ()  [unwired: 9 in]
                  }
                }
              }
            }
          }
          event "EnableJoystick": Value Change {
            n228 = event-data() -> ()  [unwired: 1 in, 6 out]
            n229 = case shown="True" "EnableJoystick" {
              frame False {
              }
              frame True {
                n230 = call "ReturnToJoystick.vi"() -> ()  [unwired: 12 in]
              }
            }
          }
          event "resetcontact": Value Change {
            n231 = event-data() -> ()  [unwired: 1 in, 6 out]
            n232 = case shown="True" "resetcontact" {
              tunnel: w329 -> [_ w334]
              frame False {
              }
              frame True {
                n233 = call "VXM_MotorPositionF.vi"() -> ("Position"=w343:i32[])  [unwired: 11 in]
                n234 = local write "In Contact"(FALSE ("In Contact")) -> ()
                n235 = Index Array(array=w343, index=2) -> (element=w341:i32)
                n236 = Add(x=-3000, y=w341) -> (x+y=w338:i32)
                n237 = call "StatusGood.vi"("Text.Text"="Please reset position 1") -> ()  [unwired: 11 in]
                n238 = Unbundle By Name(w334) -> ("ControlRefs.WaferAlignment"=w335:refnum<vi>)
                n239 = local read "Position 1"() -> (w339:i32[])
                n240 = property class="Clust (strict)"(reference=w335) -> ("Value"=w333:T1)  [unwired: 1 in, 2 out]
                n241 = Replace Array Subset(array=w339, new element=w338, index=2) -> (w332:i32[])
                n242 = local write "Position 1"(w332) -> ()
                n243 = Bundle By Name(cluster=w333, "Position 1"=w332) -> (w331:T1)
                n244 = local write "WaferAlignment"(w331) -> ()
              }
            }
          }
          event "Position 3": Value Change {
            # "Move to position 3"
            n245 = event-data() -> ()  [unwired: 1 in, 6 out]
            n246 = local read "In Contact"() -> (w348:bool)
            n247 = call "MovePos3.vi"("In Contact in"=w348, "Position 3"="Position 3", "UiDefinition 2"=w345) -> ("In Contact out"=w347:bool)  [unwired: 8 in]
            n248 = local write "In Contact"(w347) -> ()
          }
          event "Align Position 3": Value Change {
            n249 = event-data() -> ()  [unwired: 1 in, 6 out]
            n250 = case shown="True" "Align Position 3" {
              tunnel: w349 -> [_ w353]
              frame False {
              }
              frame True {
                n251 = call "VXM_MotorPositionF.vi"() -> ("Position"=w351:i32[])  [unwired: 11 in]
                "Position 3" <- w351
                n252 = control-ref of="Align Position 3"() -> (w357:refnum<vi>)
                n253 = property class="Bool"(reference=w357, "Colors [4]"=cluster{u32, u32}[] [{13816530, 13816530}]) -> ()  [unwired: 1 in, 2 out]
                n254 = Unbundle By Name(w353) -> ("ControlRefs.WaferAlignment"=w355:refnum<vi>)
                n255 = property class="Clust (strict)"(reference=w355) -> ("Value"=w354:T1)  [unwired: 1 in, 2 out]
                n256 = Bundle By Name(cluster=w354, "Position 3"=w351) -> (w352:T1)
                n257 = local write "WaferAlignment"(w352) -> ()
                n258 = call "StatusGood.vi"("Text.Text"="Please return to position 1 and run cycle" ("Status")) -> ()  [unwired: 11 in]
              }
            }
          }
          event "ClearPositions": Value Change {
            n259 = event-data() -> ()  [unwired: 1 in, 6 out]
            n260 = case shown="True" "ClearPositions" {
              tunnel: w359 -> [_ w366]
              frame False {
              }
              frame True {
                w362 = cluster{u32, u32}[] [{16741120, 16741120}] ("Colors [4]")
                w361 = i32[] [] ("Position 3")
                n261 = control-ref of="Align Position 1"() -> (w363:refnum<vi>)
                n262 = control-ref of="Align Position 3"() -> (w367:refnum<vi>)
                n263 = property class="Bool"(reference=w367, "Colors [4]"=w362) -> ()  [unwired: 1 in, 2 out]
                n264 = control-ref of="Align Position 2"() -> (w364:refnum<vi>)
                n265 = Unbundle By Name(w366) -> ("ControlRefs.WaferAlignment"=w365:refnum<vi>)
                n266 = property class="Bool"(reference=w364, "Colors [4]"=w362) -> ()  [unwired: 1 in, 2 out]
                n267 = property class="Bool"(reference=w363, "Colors [4]"=w362) -> ()  [unwired: 1 in, 2 out]
                n268 = property class="Clust (strict)"(reference=w365) -> ("Value"=w369:T1)  [unwired: 1 in, 2 out]
                n269 = local write "Position 3"(w361) -> ()
                n270 = local write "Position 2"(w361) -> ()
                n271 = local write "Position 1"(w361) -> ()
                n272 = Bundle By Name(cluster=w369, "Position 3"=w361, "Position 1"=w361, "Position 2"=w361) -> (w368:T1)
                n273 = local write "WaferAlignment"(w368) -> ()
                n274 = call "StatusGood.vi"("Text.Text"="Please set position 1" ("Status")) -> ()  [unwired: 11 in]
              }
            }
          }
          event "Align Position 2": Value Change {
            # "Set Align to Position 2"
            n275 = event-data() -> ()  [unwired: 1 in, 6 out]
            n276 = case shown="True" "Align Position 2" {
              tunnel: w371 -> [_ w376]
              frame False {
              }
              frame True {
                n277 = Unbundle By Name(w376) -> ("Microsites"=w380:refnum<k24>)
                n278 = call "VXM_MotorPositionF.vi"() -> ("Position"=w377:i32[])  [unwired: 11 in]
                "Position 2" <- w377
                n279 = local read "Steps Per micron"() -> (w383:dbl)
                n280 = local read "Chip Orientation"() -> (w382:i32)
                n281 = control-ref of="Align Position 2"() -> (w384:refnum<vi>)
                n282 = local read "Position 1"() -> (w385:i32[])
                n283 = call "AlignPosition2.vi"("Chip Orientation"=w382, "Steps Per micron"=w383, "Position 1"=w385, "Microsites"=w380, "Boolean in"=w384) -> ("Array"=w373:dbl[], "Numeric"=w374:dbl)  [unwired: 5 in]
                n284 = Unbundle By Name(w376) -> ("ControlRefs.WaferAlignment"=w379:refnum<vi>)
                n285 = local write "Scale Misalign"(w374) -> ()
                n286 = local write "Rotation Misalign"(w373) -> ()
                n287 = property class="Clust (strict)"(reference=w379) -> ("Value"=w378:T1)  [unwired: 1 in, 2 out]
                n288 = Bundle By Name(cluster=w378, "Position 2"=w377, "Scale Misalign"=w374, "Rotation Misalign"=w373) -> (w375:T1)
                n289 = call "StatusGood.vi"("Text.Text"="Please return to position 1 and run cycle" ("Status")) -> ()  [unwired: 11 in]
                n290 = local write "WaferAlignment"(w375) -> ()
              }
            }
          }
        }
        "UiDefinition 3" <- w182
      }
    }
    frame #6 {
      # "Close all tools"
      n291 = local read "VISA resource name"() -> (w387:refnum<visa-resource-name>)
      n292 = flat-sequence {
        frame #0 {
          n293 = call "Vxmdriverlv8.Vi"("Chars to send"="Q") -> ()  [unwired: 21 in, 6 out]
        }
        frame #1 {
          n294 = call "Vxmdriverlv8.Vi"("Close Port"=TRUE) -> ()  [unwired: 21 in, 6 out]
        }
      }
      n295 = call "Close.vi"("VISA resource name"=w387) -> ("error out"=w388:errorcluster)  [unwired: 10 in]
      n296 = call <vilib>:"Simple Error Handler.vi"("error in (no error)"=w388) -> ()  [unwired: 4 in, 5 out]
    }
  }
  n297 = case shown="True" w1 {
    frame False {
    }
    frame True {
      n298 = Stop(stop? (T)=TRUE) -> ()
    }
  }
